vi "Drive TeleOp.vi"(11 "Controller Values":T1) -> ()   [LabVIEW 2018]
uses:
  Support Code/Controller Values.ctl
  Framework/Robot Global Data.vi
  <vilib>/Rock Robotics/Network Tables/NT Write Numeric Array.vi
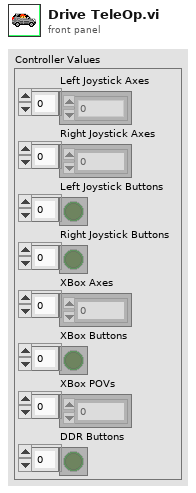
[diagram p1: front panel]
types:
  T1 = typedef "Controller Values.ctl" = cluster{"Left Joystick Axes ":dbl[], "Right Joystick Axes":dbl[], "Left Joystick Buttons":bool[], "Right Joystick Buttons":bool[], "XBox Axes":dbl[], "XBox Buttons":bool[], "XBox POVs":i16[], "DDR Buttons":bool[]}
  T2 = typedef "WPI_MotorControlDeviceRef.ctl" = cluster{"DeviceStatus":errorcluster, "Type":T3, "PWM":cluster{"PWM Channel":T4, "DeadBand":T5}, "CAN":cluster{"Device Number":u8, "SetOutput VI Ref":variant, "GetOutput VI Ref":variant, "Enable VI Ref":variant, "Disable VI Ref":variant, "Data":variant}, "Invert":bool, "DIO PWM":cluster{"PWM \"Enable\" Channel":T4, "DIOChannel":T6, "PWM Rate":dbl}}
  T3 = typedef "WPI_MotorControlType.ctl" = enum16{"PWM", "CAN", "DIO PWM"}
  T4 = typedef "FPGA_DIOPWMChannel.ctl" = enum8{"PWM 0", "PWM 1", "PWM 2", "PWM 3", "PWM 4", "PWM 5", "PWM 6", "PWM 7", "PWM 8", "PWM 9", "PWM MXP 0", "PWM MXP 1", "PWM MXP 2", "PWM MXP 3", "PWM MXP 4", "PWM MXP 5", "PWM MXP 6", "PWM MXP 7", "PWM MXP 8", "PWM MXP 9", "Invalid"}
  T5 = typedef "WPI_PWMDeadband.ctl" = cluster{"Name":string, "maxPositivePwm":i32, "minPositivePwm":i32, "centerPwm":i32, "maxNegativePwm":i32, "minNegativePwm":i32, "angularRange":u16}
  T6 = typedef "FPGA_DIOChannel.ctl" = enum8{"DIO 0", "DIO 1", "DIO 2", "DIO 3", "DIO 4", "DIO 5", "DIO 6", "DIO 7", "DIO 8", "DIO 9", "DIO MXP 0", "DIO MXP 1", "DIO MXP 2", "DIO MXP 3", "DIO MXP 4", "DIO MXP 5", "DIO MXP 6", "DIO MXP 7", "DIO MXP 8", "DIO MXP 9", "DIO MXP 10", "DIO MXP 11", "DIO MXP 12", "DIO MXP 13", "DIO MXP 14", "DIO MXP 15", "SPI Port CS1", "SPI Port CS2", "SPI Port CS3", "SPI Port MISO", "SPI Port MOSI", "Invalid"}
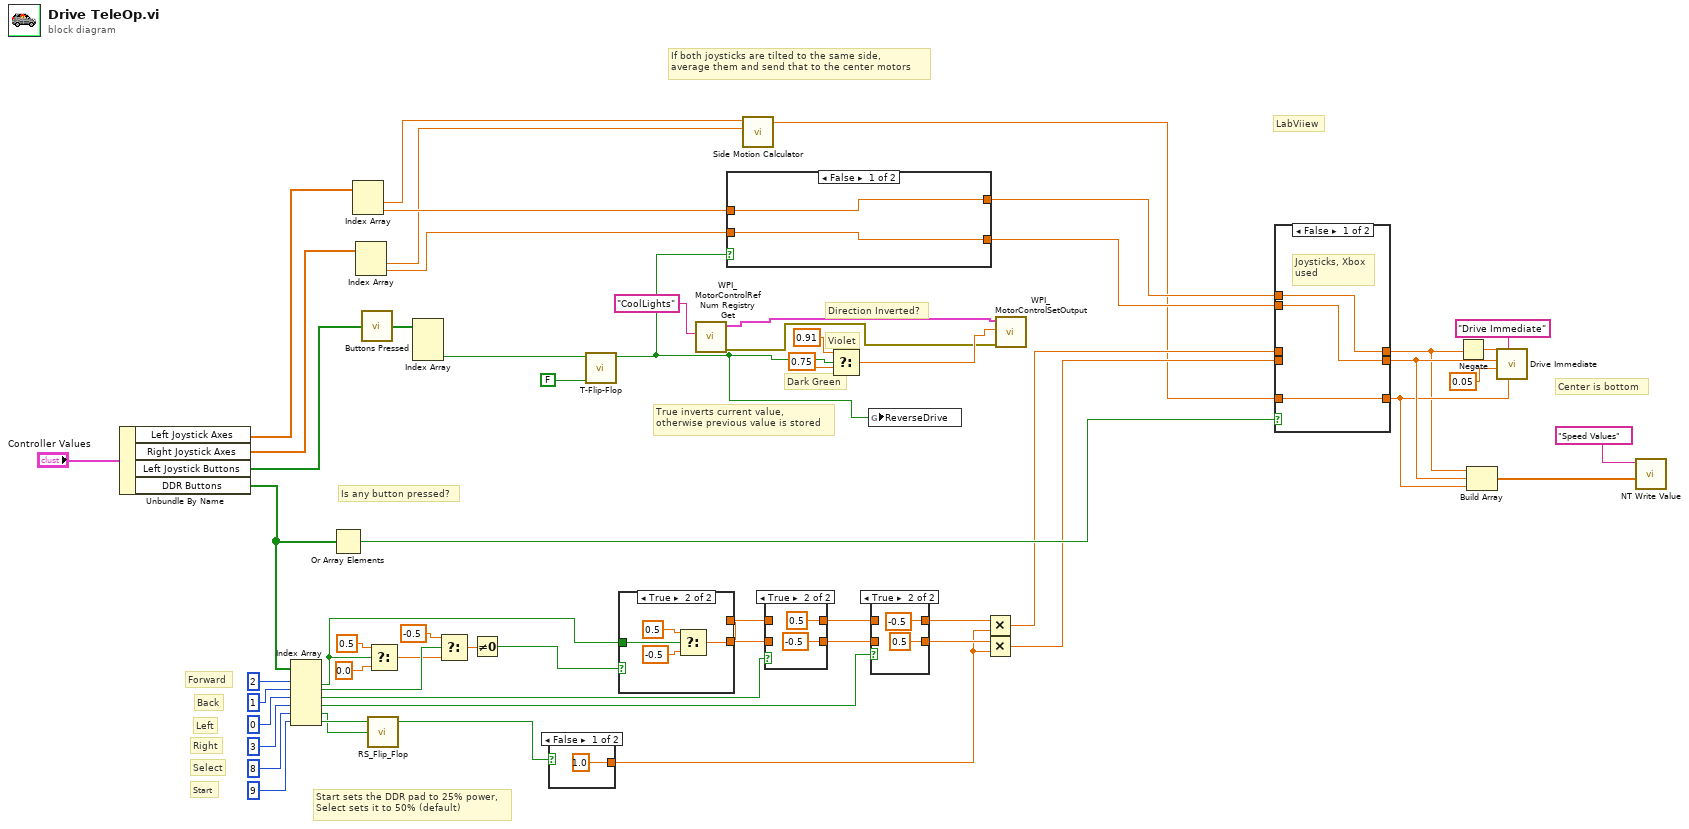
[diagram p0: block diagram]
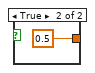
[diagram p2: hidden frame]
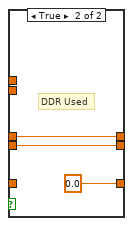
[diagram p3: hidden frame]
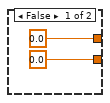
[diagram p6: hidden frame]
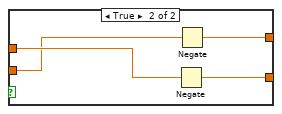
[diagram p7: hidden frame]
diagram:
  # "Dark Green"
  # "Violet"
  # "True inverts current value,\notherwise previous value is stored"
  # "If both joysticks are tilted to the same side,\naverage them and send that to the center motors"
  # "Start sets the DDR pad to 25% power,\nSelect sets it to 50% (default)"
  # "Center is bottom"
  # "Is any button pressed?"
  # "LabViiew"
  # "Start"
  # "Select"
  # "Right"
  # "Left"
  # "Back"
  # "Forward"
  # "Direction Inverted?"
  n1 = Unbundle By Name("Controller Values") -> ("Left Joystick Axes"=w16:dbl[], "Right Joystick Axes"=w15:dbl[], "Left Joystick Buttons"=w14:bool[], "DDR Buttons"=w13:bool[])
  n2 = Index Array(array=w13, index #1=2 ("index"), index #2=1 ("index"), index #3=0 ("index"), index #4=3 ("index"), index #5=8 ("index"), index #6=9 ("index")) -> (element #1=w23:bool, element #2=w50:bool, element #3=w46:bool, element #4=w43:bool, element #5=w35:bool, element #6=w36:bool)
  n3 = Or Array Elements(Boolean array=w13) -> (logical OR=w37:bool)
  n4 = Index Array(array=w16) -> (element #1=w20:dbl, element #2=w22:dbl)  [unwired: 2 in]
  n5 = Index Array(array=w15) -> (element #1=w19:dbl, element #2=w21:dbl)  [unwired: 2 in]
  n6 = call "Buttons Pressed.vi"("Button Values"=w14) -> ("Button Presses"=w24:bool[])
  n7 = call "RS_Flip_Flop.vi"("Set"=w35, "Reset"=w36) -> ("Q"=w34:bool)  [unwired: 1 in, 2 out]
  n8 = Select(t=0.5, s=w23, f=0.0) -> (s? t:f=w49:dbl)
  n9 = Index Array(array=w24) -> (element #3=w11:bool)  [unwired: 3 in, 2 out]
  n10 = Select(t=-0.5, s=w50, f=w49) -> (s? t:f=w47:dbl)
  n11 = Not Equal To 0?(x=w47) -> (x != 0?=w38:bool)
  n12 = case shown="False" w34 {
    tunnel: [1.0 0.5] -> w30
    frame False {
    }
    frame True {
    }
  }
  n13 = call "T-Flip-Flop.vi"("Starting Value"=FALSE, "Flip"=w11) -> ("Value"=w4:bool)  [unwired: 9 in]
  n14 = case shown="True" w38 {
    tunnel: [0.0 w64] -> w45
    tunnel: [0.0 w64] -> w44
    tunnel: w23 -> [_ w67]
    frame False {
    }
    frame True {
      n15 = Select(t=0.5, s=w67, f=-0.5) -> (s? t:f=w64:dbl)
    }
  }
  n16 = call <vilib>:"WPI_MotorControlRefNum Registry Get.vi"("refnum name"="CoolLights") -> ("error out"=w5:errorcluster, "MotorControlDevRef"=w7:T2)  [unwired: 9 in]
  n17 = case shown="False" w4 {
    tunnel: w22 -> [w69 w73]
    tunnel: w21 -> [w68 w71]
    tunnel: [w69 w70] -> w40
    tunnel: [w68 w72] -> w39
    frame False {
    }
    frame True {
      n18 = Negate(x=w73) -> (-x=w72:dbl)
      n19 = Negate(x=w71) -> (-x=w70:dbl)
    }
  }
  n20 = call "Side Motion Calculator.vi"("Numeric 2"=w19, "Numeric"=w20) -> ("Numeric 3"=w18:dbl)  [unwired: 8 in, 1 out]
  n21 = case shown="True" w46 {
    tunnel: [w75 0.5] -> w42
    tunnel: w45 -> [w75 _]
    tunnel: w44 -> [w74 _]
    tunnel: [w74 -0.5] -> w41
    frame False {
    }
    frame True {
    }
  }
  n22 = Select(t=0.91, s=w4, f=0.75) -> (s? t:f=w8:dbl)
  n23 = global write "Robot Global Data.vi" "ReverseDrive"(w4) -> ()
  n24 = case shown="True" w43 {
    tunnel: w42 -> [w79 _]
    tunnel: [w79 -0.5] -> w33
    tunnel: w41 -> [w78 _]
    tunnel: [w78 0.5] -> w31
    frame False {
    }
    frame True {
    }
  }
  n25 = Multiply(x=w33, y=w30) -> (x*y=w32:dbl)
  n26 = Multiply(x=w31, y=w30) -> (x*y=w29:dbl)
  n27 = call <vilib>:"WPI_MotorControlSetOutput.vi"("error in (no error)"=w5, "Output"=w8, "MotorControlDevRef"=w7) -> ()  [unwired: 6 in, 3 out]
  n28 = case shown="False" w37 {
    tunnel: w40 -> [w84 _]
    tunnel: w39 -> [w83 _]
    tunnel: [w84 w87] -> w1
    tunnel: [w83 w86] -> w26
    tunnel: w18 -> [w82 _]
    tunnel: [w82 0.0] -> w25
    tunnel: w32 -> [_ w87]
    tunnel: w29 -> [_ w86]
    frame False {
      # "Joysticks, Xbox\nused"
    }
    frame True {
      # "DDR Used"
    }
  }
  n29 = Negate(x=w1) -> (-x=w2:dbl)
  n30 = Build Array(w1, w26, w25) -> (w28:dbl[])
  n31 = call "Drive Immediate.vi"("Center Setpoint"=w25, "Description"="Drive Immediate", "Deadband Value"=0.05, "Right Setpoint"=w26, "Left Setpoint"=w2) -> ()  [unwired: 6 in, 1 out]
  n32 = call-poly <vilib>:"NT Write Value.vi"("Numeric Array"=w28, "Name"="Speed Values") -> ()  [unwired: 9 in, 1 out]
